vi "Global 1.vi"() -> ()   [LabVIEW 2020]
panel:
  in  "Sincrono":bool
  in  "apagar":bool
  in  "modular":bool
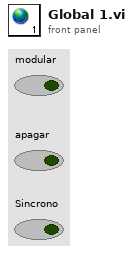
[diagram p1: front panel]
diagram:
